vi "TestingStraight.vi"() -> ()   [LabVIEW 2016]
uses:
  <vilib>/Rock Robotics/WPI/Utilities/WPI_GetSetVariantRefNum.vi
panel:
  in  "Zero Yaw":bool
  in  "Config":T1={"Distance"=100.0, "MaxVelocity"=60.0, "MaxAccel"=50.0, "InitialVelocity"=0.0, "FinalVelocity"=0.0}
  out "Outputs":cluster{dbl, dbl, "Turn":dbl}(graph)
  in  "Go":bool
  in  "Go Backwards":bool
  out "Vel":cluster{dbl, "vel":dbl}(graph)
  out "Pos":cluster{dbl, "pos":dbl}(graph)={50.0, "pos"=48.31556625}
  in  "Linear Constants":T2={"FF"=0.0066, "AFF"=0.0018, "PID gains"={"P"=0.07, "I"=0.0, "D"=0.0}} {"PID gains"."D" format="%.3f"; "PID gains"."I" format="%.3f"; "PID gains"."P" format="%.3f"}
  # "MAKE DEFAULT"
  # ".009"
  # ".002"
  # ".07"
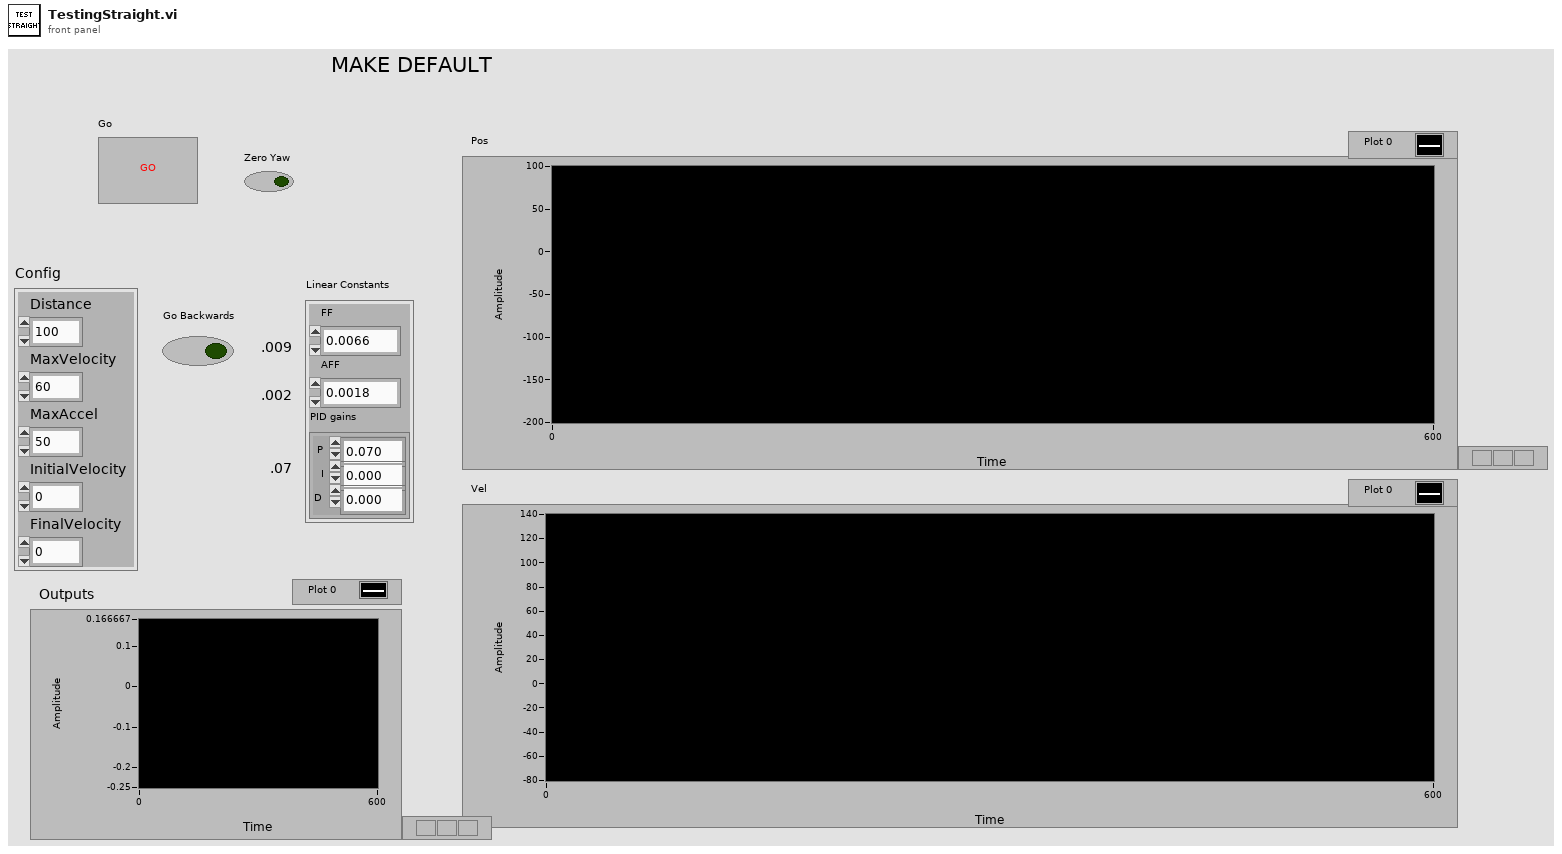
[diagram p1: front panel]
types:
  T1 = cluster{"Distance":dbl, "MaxVelocity":dbl, "MaxAccel":dbl, "InitialVelocity":dbl, "FinalVelocity":dbl}
  T2 = cluster{"FF":dbl, "AFF":dbl, "PID gains":cluster{"P":dbl, "I":dbl, "D":dbl}}
  T3 = typedef "WPI_EncoderDevRef.ctl" = cluster{"DevStatus":errorcluster, "EncoderIndex":T4, "CounterIndex":T5, "DistancePerCount":dbl, "Decoding Type":T6}
  T4 = typedef "FPGA_EncoderIdx.ctl" = enum8{"Enc 0", "Enc 1", "Enc 2", "Enc 3", "Enc 4", "Enc 5", "Enc 6", "Enc 7", "Invalid"}
  T5 = typedef "FPGA_CounterCtrSystemIndex.ctl" = enum8{"Ctr 0", "Ctr 1", "Ctr 2", "Ctr 3", "Ctr 4", "Ctr 5", "Ctr 6", "Ctr 7", "Invalid"}
  T6 = typedef "WPI_EncoderType.ctl" = enum16{"1x", "2x", "4x"}
  T7 = typedef "WPI_RobotDriveDevRef.ctl" = cluster{"DevStatus":errorcluster, "Motors[]":T8[], "Square Inputs":bool, "Max Output":dbl}
  T8 = typedef "WPI_MotorControlDeviceRef.ctl" = cluster{"DeviceStatus":errorcluster, "Type":T9, "PWM":cluster{"PWM Channel":T10, "DeadBand":T11}, "CAN":cluster{"Device Number":u8, "SetOutput VI Ref":variant, "GetOutput VI Ref":variant, "Enable VI Ref":variant, "Disable VI Ref":variant, "Data":variant}, "Invert":bool}
  T9 = typedef "WPI_MotorControlType.ctl" = enum16{"PWM", "CAN"}
  T10 = typedef "FPGA_DIOPWMChannel.ctl" = enum8{"PWM 0", "PWM 1", "PWM 2", "PWM 3", "PWM 4", "PWM 5", "PWM 6", "PWM 7", "PWM 8", "PWM 9", "PWM MXP 0", "PWM MXP 1", "PWM MXP 2", "PWM MXP 3", "PWM MXP 4", "PWM MXP 5", "PWM MXP 6", "PWM MXP 7", "PWM MXP 8", "PWM MXP 9", "Invalid"}
  T11 = typedef "WPI_PWMDeadband.ctl" = cluster{"Name":string, "maxPositivePwm":i32, "minPositivePwm":i32, "centerPwm":i32, "maxNegativePwm":i32, "minNegativePwm":i32, "angularRange":u16}
  T12 = cluster{dbl, "distance/rotation":dbl, "distance/rotation":dbl}
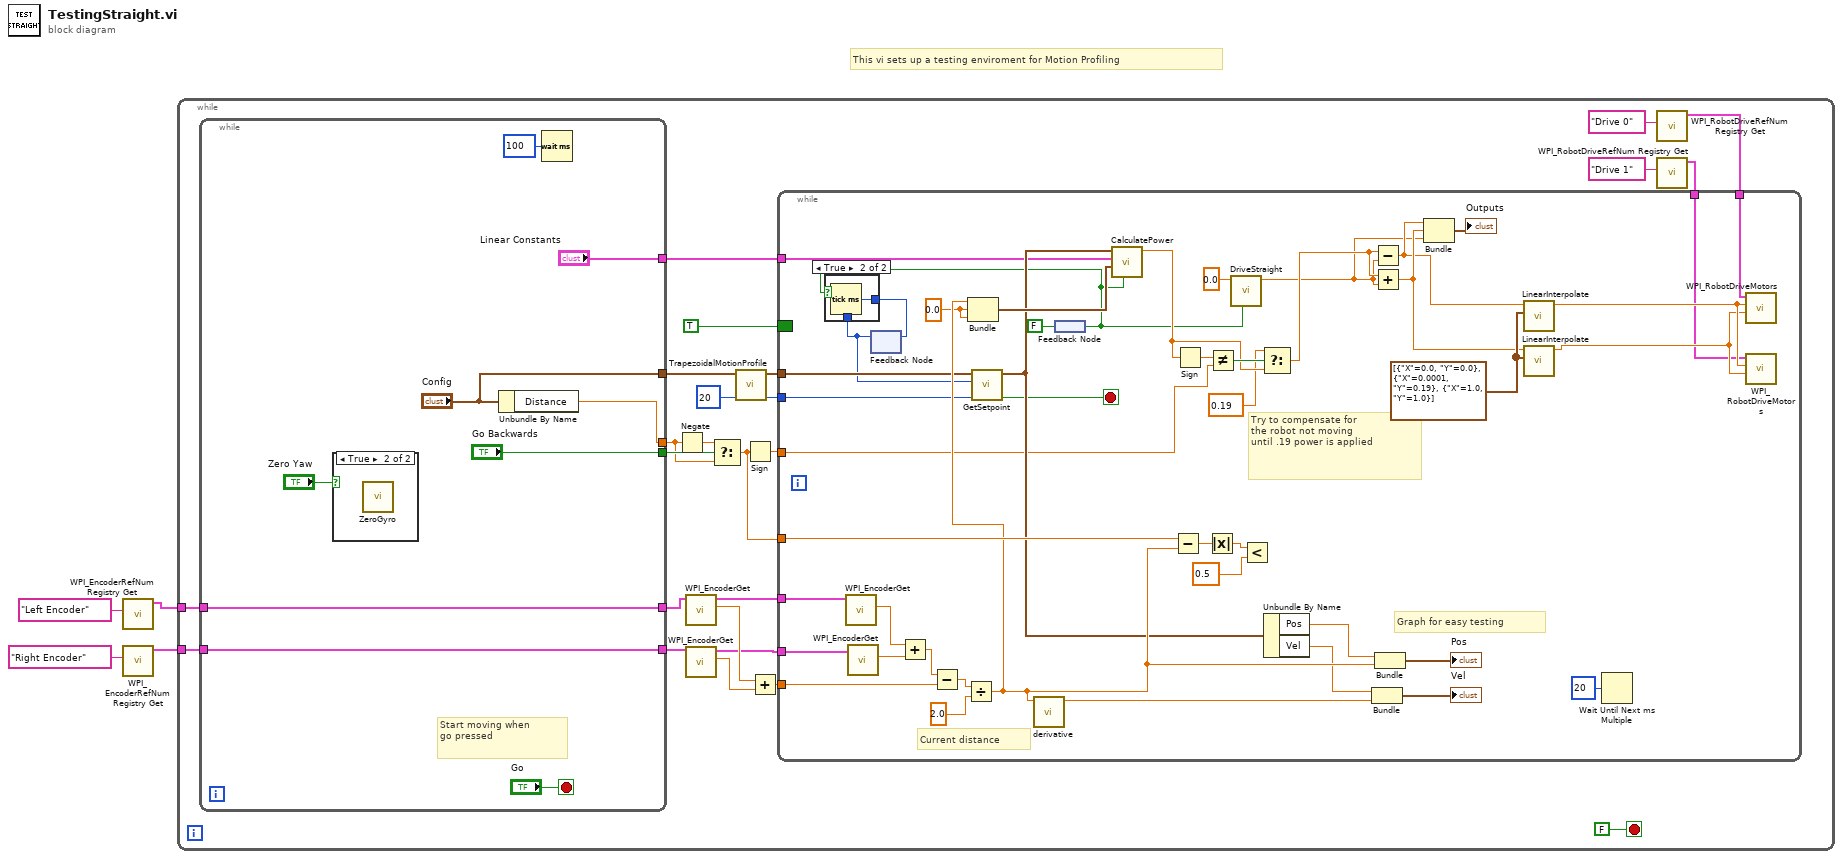
[diagram p0: block diagram]
diagram:
  # "This vi sets up a testing enviroment for Motion Profiling"
  n1 = call <vilib>:"WPI_EncoderRefNum Registry Get.vi"("refnum name"="Left Encoder") -> ("EncoderDevRef"=w2:T3)  [unwired: 9 in, 1 out]
  n2 = call <vilib>:"WPI_EncoderRefNum Registry Get.vi"("refnum name"="Right Encoder") -> ("EncoderDevRef"=w1:T3)  [unwired: 9 in, 1 out]
  n3 = while {
    tunnel: w2 -> [w12]
    tunnel: w1 -> [w11]
    stop <- FALSE stop-if-true
    n4 = while {
      tunnel: ["Go Backwards"] -> w14
      tunnel: w12 -> [w35]
      tunnel: [w35] -> w13
      tunnel: w11 -> [w34]
      tunnel: [w34] -> w10
      tunnel: [w33] -> w9
      tunnel: ["Config"] -> w8
      tunnel: ["Linear Constants"] -> w7
      stop <- "Go" stop-if-true
      # "Start moving when\ngo pressed"
      n5 = case shown="True" "Zero Yaw" {
        frame False {
        }
        frame True {
          n6 = call "ZeroGyro.vi"() -> ()  [unwired: 11 in, 1 out]
        }
      }
      n7 = Unbundle By Name("Config") -> ("Distance"=w33:dbl)
      n8 = Wait (ms)(milliseconds to wait=u32 100 ("millisecond multiple")) -> ()  [unwired: 1 out]
    }
    n9 = Negate(x=w9) -> (-x=w28:dbl)
    n10 = call <vilib>:"WPI_EncoderGet.vi"("EncoderDevRef"=w13) -> ("Distance"=w25:dbl, "EncoderDevRef"=w20:T3)  [unwired: 5 in, 4 out]
    n11 = call <vilib>:"WPI_EncoderGet.vi"("EncoderDevRef"=w10) -> ("Distance"=w24:dbl, "EncoderDevRef"=w19:T3)  [unwired: 5 in, 4 out]
    n12 = Select(t=w28, s=w14, f=w9) -> (s? t:f=w16:dbl)
    n13 = call "TrapezoidalMotionProfile.vi"("dt"=u32 20, "Config"=w8) -> ("dt"=w21:u32, "Profile"=w29:cluster{"Pos":dbl, "Vel":dbl, "Accel":dbl}[])  [unwired: 8 in]
    n14 = Sign(1:w16) -> (0:w15:dbl)
    n15 = Add(x=w25, y=w24) -> (x+y=w23:dbl)
    n16 = call <vilib>:"WPI_RobotDriveRefNum Registry Get.vi"("refnum name"="Drive 0") -> ("RobotDriveDevRef"=w6:T7)  [unwired: 9 in, 1 out]
    n17 = call <vilib>:"WPI_RobotDriveRefNum Registry Get.vi"("refnum name"="Drive 1") -> ("RobotDriveDevRef"=w5:T7)  [unwired: 9 in, 1 out]
    n18 = while {
      tunnel: w29 -> [w68]
      tunnel: w16 -> [w78]
      border: TRUE ("Reset") -> [_]
      tunnel: w23 -> [w73]
      tunnel: w21 -> [w67]
      tunnel: w20 -> [w60]
      tunnel: w19 -> [w59]
      tunnel: w15 -> [w57]
      tunnel: w7 -> [w49]
      tunnel: w6 -> [w46]
      tunnel: w5 -> [w45]
      stop <- w61 stop-if-true
      w44 = cluster{"X":dbl, "Y":dbl}[] [{"X"=0.0, "Y"=0.0}, {"X"=0.0001, "Y"=0.19}, {"X"=1.0, "Y"=1.0}] ("Points")
      w70 = 0.0 ("distance/rotation")
      # "Try to compensate for\nthe robot not moving\nuntil .19 power is applied"
      # "Graph for easy testing"
      # "Current distance"
      n19 = call <vilib>:"WPI_EncoderGet.vi"("EncoderDevRef"=w60) -> ("Distance"=w76:dbl)  [unwired: 5 in, 5 out]
      n20 = call <vilib>:"WPI_EncoderGet.vi"("EncoderDevRef"=w59) -> ("Distance"=w50:dbl)  [unwired: 5 in, 5 out]
      n21 = feedback #1() -> (w47:u32)  [unwired: 1 in]
      n22 = Add(x=w76, y=w50) -> (x+y=w74:dbl)
      n23 = Subtract(x=w74, y=w73) -> (x-y=w75:dbl)
      n24 = Divide(x=w75, y=2.0 ("distance/rotation")) -> (x/y=w71:dbl)
      n25 = Bundle(w71, "distance/rotation"=w70, "distance/rotation"=w70) -> (w72:T12)  [unwired: 1 in]
      n26 = call "GetSetpoint.vi"("dt"=w67, "Start Time"=w47, "Profile"=w68) -> ("Profile done?"=w61:bool, "Setpoints"=w66:cluster{"Pos":dbl, "Vel":dbl, "Accel":dbl})  [unwired: 7 in]
      n27 = call "derivative.vi"("x"=w71) -> ("dx/dt"=w77:dbl)  [unwired: 10 in]
      n28 = feedback-in #2(FALSE ("Reset")) -> ()
      n29 = feedback #2() -> (w43:bool)
      n30 = case shown="True" w43 {
        tunnel: [w85 w86] -> w48
        tunnel: w47 -> [w85 _]
        frame False {
        }
        frame True {
          n31 = Tick Count (ms)() -> (millisecond timer value=w86:u32)
        }
      }
      n32 = feedback-in #1(w48) -> ()
      n33 = call "CalculatePower.vi"("Reset"=w43, "Process Variables"=w72, "Constants"=w49, "Setpoints"=w66) -> ("Power"=w55:dbl)  [unwired: 7 in]
      n34 = Subtract(x=w78, y=w71) -> (x-y=w82:dbl)
      n35 = Sign(1:w55) -> (0:w58:dbl)
      n36 = Absolute Value(x=w82) -> (abs(x)=w81:dbl)
      n37 = Not Equal?(x=w58, y=w57) -> (x != y?=w56:bool)
      n38 = call "DriveStraight.vi"("Reset"=w43, "Angle"=0.0) -> ("Turn"=w39:dbl)  [unwired: 9 in]
      n39 = Less?(x=w81, y=0.5 ("Closeness at end")) -> ()  [unwired: 1 out]
      n40 = Select(t=0.19, s=w56, f=w55) -> (s? t:f=w53:dbl)
      n41 = Unbundle By Name(w66) -> ("Pos"=w65:dbl, "Vel"=w64:dbl)
      n42 = Bundle("Vel"=w64, "dx/dt"=w77) -> (→"Vel":cluster{"Vel":dbl, "dx/dt":dbl})  [unwired: 1 in]
      n43 = Subtract(x=w53, y=w39) -> (x-y=w40:dbl)
      n44 = Add(x=w53, y=w39) -> (x+y=w41:dbl)
      n45 = Bundle("Pos"=w65, w71) -> (→"Pos":cluster{"Pos":dbl, dbl})  [unwired: 1 in]
      n46 = Bundle(w40, w41, "Turn"=w39) -> (→"Outputs":cluster{dbl, dbl, "Turn":dbl})  [unwired: 1 in]
      n47 = call "LinearInterpolate.vi"("Points"=w44, "Value"=w40) -> ("Output"=w52:dbl)  [unwired: 9 in]
      n48 = call "LinearInterpolate.vi"("Points"=w44, "Value"=w41) -> ("Output"=w51:dbl)  [unwired: 9 in]
      n49 = Wait Until Next ms Multiple(millisecond multiple=u32 20) -> ()  [unwired: 1 out]
      n50 = call <vilib>:"WPI_RobotDriveMotors.vi"("RightSpeed"=w51, "LeftSpeed"=w52, "RobotDriveDevRef"=w46) -> ()  [unwired: 6 in, 3 out]
      n51 = call <vilib>:"WPI_RobotDriveMotors.vi"("RightSpeed"=w51, "LeftSpeed"=w52, "RobotDriveDevRef"=w45) -> ()  [unwired: 6 in, 3 out]
    }
  }
